vi "HH_AllDllFunctions_UIThread.vi"   [LabVIEW 2017]
uses:
  hhlib_x86_x64_UIThread.llb/HH_DllPath_global.vi
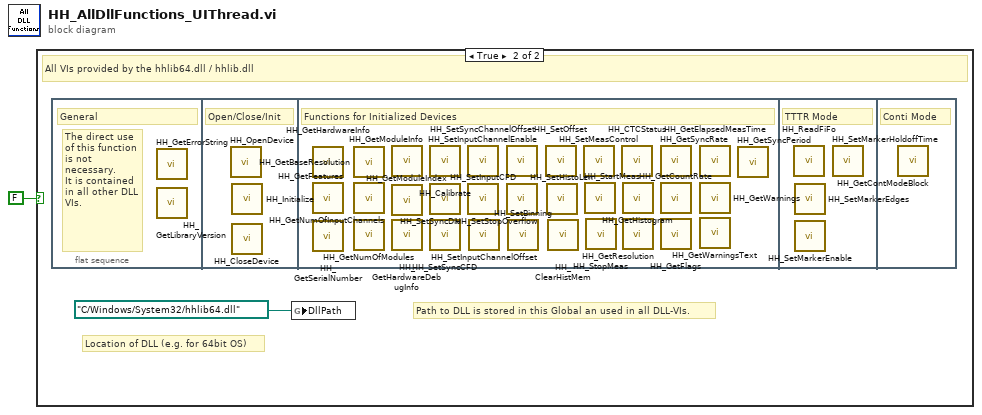
[diagram p0: block diagram]
diagram:
  n1 = case shown="True" FALSE {
    frame False {
    }
    frame True {
      # "Location of DLL (e.g. for 64bit OS)"
      # "Path to DLL is stored in this Global an used in all DLL-VIs."
      # "All VIs provided by the hhlib64.dll / hhlib.dll"
      n2 = flat-sequence {
        frame #0 {
          # "The direct use of this function is not necessary.\nIt is contained in all other DLL VIs."
          # "General"
          n3 = call "HH_GetErrorString.vi"() -> ()  [unwired: 9 in, 3 out]
          n4 = call "HH_GetLibraryVersion.vi"() -> ()  [unwired: 9 in, 3 out]
        }
        frame #1 {
          # "Open/Close/Init"
          n5 = call "HH_OpenDevice.vi"() -> ()  [unwired: 9 in, 3 out]
          n6 = call "HH_Initialize.vi"() -> ()  [unwired: 10 in, 2 out]
          n7 = call "HH_CloseDevice.vi"() -> ()  [unwired: 10 in, 2 out]
        }
        frame #2 {
          # "Functions for Initialized Devices"
          n8 = call "HH_GetHardwareInfo.vi"() -> ()  [unwired: 7 in, 5 out]
          n9 = call "HH_GetFeatures.vi"() -> ()  [unwired: 9 in, 3 out]
          n10 = call "HH_GetSerialNumber.vi"() -> ()  [unwired: 9 in, 3 out]
          n11 = call "HH_GetBaseResolution.vi"() -> ()  [unwired: 8 in, 4 out]
          n12 = call "HH_GetNumOfInputChannels.vi"() -> ()  [unwired: 9 in, 3 out]
          n13 = call "HH_GetNumOfModules.vi"() -> ()  [unwired: 9 in, 3 out]
          n14 = call "HH_GetModuleInfo.vi"() -> ()  [unwired: 8 in, 4 out]
          n15 = call "HH_GetModuleIndex.vi"() -> ()  [unwired: 9 in, 3 out]
          n16 = call "HH_GetHardwareDebugInfo.vi"() -> ()  [unwired: 9 in, 3 out]
          n17 = call "HH_Calibrate.vi"() -> ()  [unwired: 10 in, 2 out]
          n18 = call "HH_SetSyncDiv.vi"() -> ()  [unwired: 10 in, 2 out]
          n19 = call "HH_SetSyncCFD.vi"() -> ()  [unwired: 10 in, 2 out]
          n20 = call "HH_SetSyncChannelOffset.vi"() -> ()  [unwired: 10 in, 2 out]
          n21 = call "HH_SetInputCFD.vi"() -> ()  [unwired: 10 in, 2 out]
          n22 = call "HH_SetInputChannelOffset.vi"() -> ()  [unwired: 10 in, 2 out]
          n23 = call "HH_SetInputChannelEnable.vi"() -> ()  [unwired: 10 in, 2 out]
          n24 = call "HH_SetStopOverflow.vi"() -> ()  [unwired: 10 in, 2 out]
          n25 = call "HH_SetBinning.vi"() -> ()  [unwired: 10 in, 2 out]
          n26 = call "HH_SetOffset.vi"() -> ()  [unwired: 10 in, 2 out]
          n27 = call "HH_SetHistoLen.vi"() -> ()  [unwired: 9 in, 3 out]
          n28 = call "HH_ClearHistMem.vi"() -> ()  [unwired: 10 in, 2 out]
          n29 = call "HH_SetMeasControl.vi"() -> ()  [unwired: 10 in, 2 out]
          n30 = call "HH_StartMeas.vi"() -> ()  [unwired: 10 in, 2 out]
          n31 = call "HH_StopMeas.vi"() -> ()  [unwired: 10 in, 2 out]
          n32 = call "HH_CTCStatus.vi"() -> ()  [unwired: 9 in, 3 out]
          n33 = call "HH_GetHistogram.vi"() -> ()  [unwired: 9 in, 3 out]
          n34 = call "HH_GetResolution.vi"() -> ()  [unwired: 9 in, 3 out]
          n35 = call "HH_GetSyncRate.vi"() -> ()  [unwired: 9 in, 3 out]
          n36 = call "HH_GetCountRate.vi"() -> ()  [unwired: 9 in, 3 out]
          n37 = call "HH_GetFlags.vi"() -> ()  [unwired: 9 in, 3 out]
          n38 = call "HH_GetElapsedMeasTime.vi"() -> ()  [unwired: 9 in, 3 out]
          n39 = call "HH_GetWarnings.vi"() -> ()  [unwired: 9 in, 3 out]
          n40 = call "HH_GetWarningsText.vi"() -> ()  [unwired: 9 in, 3 out]
          n41 = call "HH_GetSyncPeriod.vi"() -> ()  [unwired: 9 in, 3 out]
        }
        frame #3 {
          # "TTTR Mode"
          n42 = call "HH_ReadFiFo.vi"() -> ()  [unwired: 8 in, 4 out]
          n43 = call "HH_SetMarkerEdges.vi"() -> ()  [unwired: 10 in, 2 out]
          n44 = call "HH_SetMarkerEnable.vi"() -> ()  [unwired: 10 in, 2 out]
          n45 = call "HH_SetMarkerHoldoffTime.vi"() -> ()  [unwired: 10 in, 2 out]
        }
        frame #4 {
          # "Conti Mode"
          n46 = call "HH_GetContModeBlock.vi"() -> ()  [unwired: 8 in, 4 out]
        }
      }
      n47 = global write "HH_DllPath_global.vi" "DllPath"(path "C:/Windows/System32/hhlib64.dll" ("DllPath")) -> ()
    }
  }
